vi "FTW-Actor-Initialized.vi"(0 "FTW Actor Instance":refnum<class "FTW-TestStep-Base.lvclass">, 5 "Initialized Response":string="{}", 9 "Positive Init?":string, 11 "error in":errorcluster) -> (4 "FTW Actor Instance out":refnum<class "FTW-TestStep-Base.lvclass">, 15 "error out":errorcluster)   [LabVIEW 2018, in "FTW-TestStep-Base.lvclass"]
uses:
  FTW-TestStep-Base.lvclass
  JSON/FTW-JSON-JoinMode.ctl
  FTW-TestStep-Base.lvclass/FTW-TestStep-Base.ctl
  526e194f-cf81-4b7c-98a1-0429ebb1b9dc.vi
  526e194f-cf81-4b7c-98a1-0429ebb1b9dc.vi/4105eb51-51f7-48d3-82bd-d64f3cda0aaf.vi
  container/FTW-Container-FromVariant.vi
  container/FTW-Container-New-FromContainer.vi
  JSON/FTW-JSON-SerializeAndDestroy.vi
  Instance/FTW-ActorInstance.lvclass
panel:
  # "Inputs"
  # "Outputs"
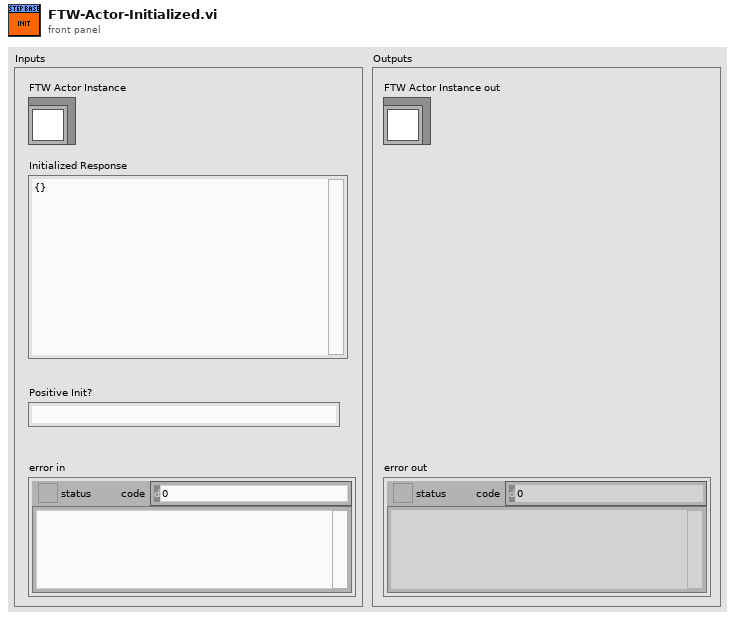
[diagram p1: front panel]
types:
  T1 = typedef "FTW-JSON-JoinMode.ctl" = enum32{"Upsert", "Update Only", "Insert Only"}
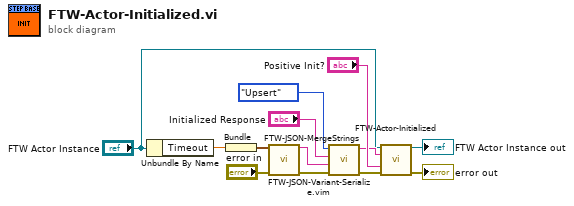
[diagram p0: block diagram]
diagram:
  n1 = Unbundle By Name("FTW Actor Instance") -> ("Timeout"=w3:dbl)
  n2 = Bundle("Timeout"=w3) -> (w4:cluster{"Timeout":dbl})  [unwired: 1 in]
  n3 = call "FTW-JSON-Variant-Serialize.vim"("Variant"=w4, "error in"="error in") -> ("JSON String"=w7:string, "error out"=w8:errorcluster)  [unwired: 12 in]
  n4 = call "FTW-JSON-MergeStrings.vi"("error in (no error)"=w8, "Initial JSON String (\"\")"=w7, "JSON string to merge (\"\")"="Initialized Response", "Update Mode (0: Upsert)"=FTW-JSON-JoinMode."Upsert") -> ("error out"=w10:errorcluster, "Merged JSON String (UTF-8)"=w9:string)  [unwired: 6 in]
  n5 = call-parent "FTW-Actor-Initialized.vi"("FTW Actor Instance"="FTW Actor Instance", "Initialized Response"=w9, "Positive Init?"="Positive Init?", "error in"=w10) -> ("FTW Actor Instance out"=→"FTW Actor Instance out":refnum<class "FTW-TestStep-Base.lvclass">, "error out"=→"error out":errorcluster)  [unwired: 10 in]
